vi "Select Level UI.vi"() -> (2 "Cancelled?":bool, 3 "Selected Level":string)   [LabVIEW 2020, in "App.lvlib" / "MazeUI.lvclass"]
uses:
  MazeUI.lvclass
  Maze/MazeGen/MazeGen.lvclass
panel:
  in  "Cancel":bool
  in  "Ok":bool
  in  "Level":i32(listbox)
  # "Select maze level:"
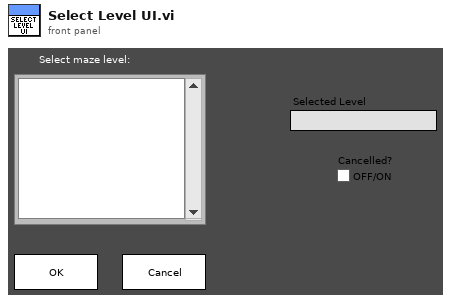
[diagram p1: front panel]
types:
  T1 = enum32{"Invalid", "Standard", "Closed", "Hidden", "Minimized", "Maximized"}
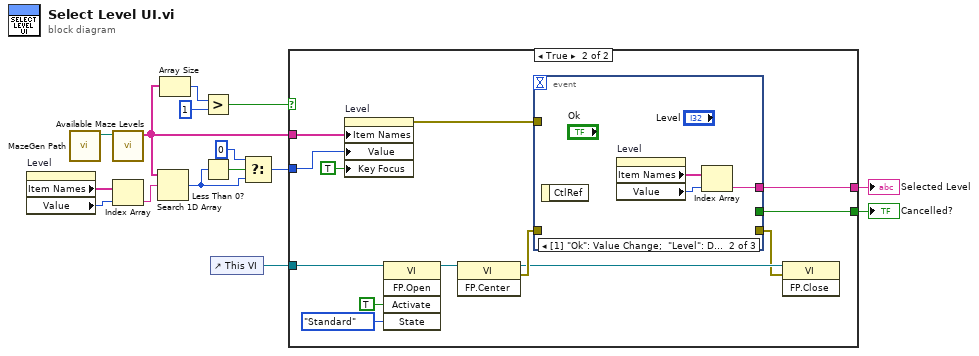
[diagram p0: block diagram]
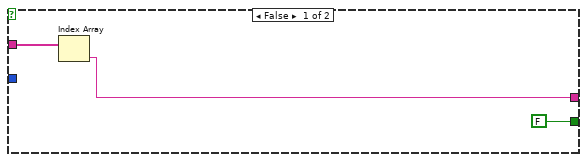
[diagram p2: hidden frame]
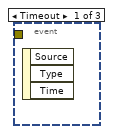
[diagram p3: hidden frame]
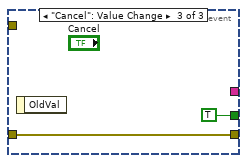
[diagram p4: hidden frame]
diagram:
  n1 = property on="Level" class="LstBox (strict)"() -> ("Item Names"=w15:string[], "Value"=w14:i32)  [unwired: 2 in, 2 out]
  n2 = call "MazeGen Path.vi"() -> ("MazeGen Path"=w1:path)  [unwired: 11 in]
  n3 = call "Available Maze Levels.vi"("MazeGen Folder"=w1) -> ("Available Maze Levels"=w6:string[])  [unwired: 10 in]
  n4 = Index Array(array=w15, index=w14) -> (element=w13:string)
  n5 = Search 1D Array(1D array=w6, element=w13) -> (index of element=w11:i32)  [unwired: 1 in]
  n6 = Array Size(array=w6) -> (size(s)=w5:i32)
  n7 = Greater?(x=w5, y=1) -> (0:w3:bool)
  n8 = Less Than 0?(x=w11) -> (x < 0?=w12:bool)
  n9 = control-ref of="This VI"() -> (w2:refnum<vi>)
  n10 = Select(t=0, s=w12, f=w11) -> (s? t:f=w9:i32)
  n11 = case shown="True" w3 {
    tunnel: w9 -> [_ w31]
    tunnel: [w17 w28] -> w8
    tunnel: [FALSE w27] -> w7
    tunnel: w6 -> [w18 w26]
    tunnel: w2 -> [_ w25]
    frame False {
      n12 = Index Array(array=w18) -> (element=w17:string)  [unwired: 1 in]
    }
    frame True {
      n13 = property on="Level" class="LstBox (strict)"("Item Names"=w26, "Value"=w31, "Key Focus"=TRUE) -> (error out=w29:errorcluster)  [unwired: 2 in, 1 out]
      n14 = invoke class="VI" method="FP.Open"(reference=w25, "Activate"=TRUE ("Activate?"), "State"=T1."Standard") -> (reference out=w22:refnum<vi>)  [unwired: 2 in, 4 out]
      n15 = invoke class="VI" method="FP.Center"(reference=w22) -> (reference out=w20:refnum<vi>, error out=w21:errorcluster)  [unwired: 2 in, 1 out]
      n16 = event shown="[1] \"Ok\": Value Change;  \"Level\": Double Click" {
        selector: _ -> [_ _ _]
        dyn-events: _ -> [_ _ _]
        timeout: _ -> [_ _ _]
        tunnel: w29 -> [_ _ _]
        tunnel: [_ w32 _] -> w28
        tunnel: [_ _ TRUE] -> w27
        tunnel: w21 -> [_ _ w35]
        tunnel: [_ _ w35] -> w19
        event Timeout {
          n17 = event-data() -> ()  [unwired: 1 in, 3 out]
        }
        event "Ok": Value Change; "Level": Double Click {
          n18 = event-data() -> ()  [unwired: 1 in, 1 out]
          n19 = property on="Level" class="LstBox (strict)"() -> ("Item Names"=w34:string[], "Value"=w33:i32)  [unwired: 2 in, 2 out]
          n20 = Index Array(array=w34, index=w33) -> (element=w32:string)
        }
        event "Cancel": Value Change {
          n21 = event-data() -> ()  [unwired: 1 in, 1 out]
        }
      }
      n22 = invoke class="VI" method="FP.Close"(reference=w20, error in=w19) -> ()  [unwired: 1 in, 3 out]
    }
  }
  "Selected Level" <- w8
  "Cancelled?" <- w7
